vi "Save data.vi"(0 "Display State In":T2, 5 "Data":T1, 9 "Container State":T3, 11 "error in (no error)":errorcluster) -> (4 "Display State Out":T2, 15 "error out":errorcluster)   [LabVIEW 2014, in "Graph with cursors XControl.xctl"]
uses:
  Graph with cursors XControl.xctl
  <vilib>/_xctls/Container State.ctl
  Graph with cursors State.ctl
  Graph with cursors Data.ctl
  <vilib>/_xctls/XControlSupport.lvlib
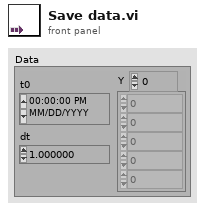
[diagram p1: front panel]
types:
  T1 = typedef "Graph with cursors XControl.xctl/Graph with cursors Data.ctl" = waveform(dbl)
  T2 = typedef "Graph with cursors XControl.xctl/Graph with cursors State.ctl" = cluster{"Cursor names":string[], "Cursor positions":dbl[], "Cursor pairs":i32, "Graph":refnum<vi>, "Prefix":string, "Base path":path}
  T3 = typedef "XControlSupport.lvlib/Container State.ctl" = cluster{"Indicator?":bool, "Run Mode?":bool, " Refnum":refnum<vi>}
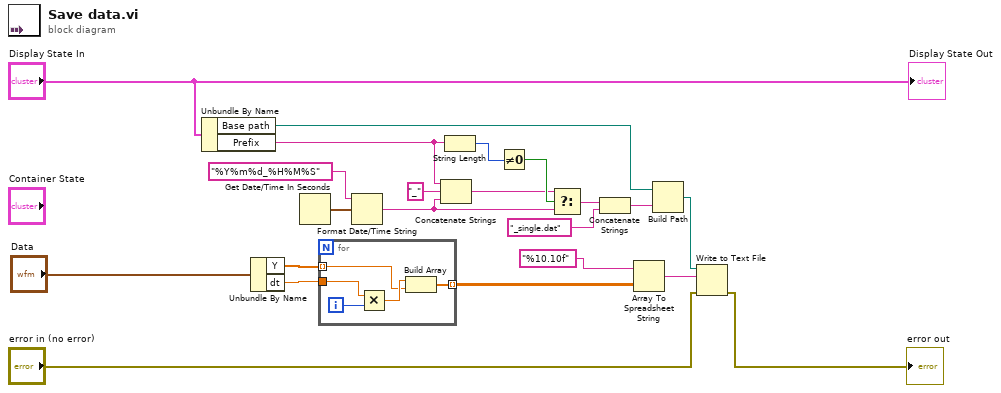
[diagram p0: block diagram]
diagram:
  n1 = Unbundle By Name("Display State In") -> ("Base path"=w11:path, "Prefix"=w10:string)
  n2 = Unbundle By Name("Data") -> ("Y"=w17:dbl[], "dt"=w16:dbl)
  n3 = Get Date/Time In Seconds() -> (seconds since 1Jan1904=w20:timestamp)
  n4 = for {
    tunnel: w17 -> [w24] mode=indexing
    tunnel: w16 -> [w26]
    tunnel: [w23] -> w1 mode=indexing
    i -> [w27]
    n5 = Multiply(x=w26, y=w27) -> (x*y=w25:dbl)
    n6 = Build Array(w25, w24) -> (w23:dbl[])
  }
  n7 = Format Date/Time String(time format string (%c)="%Y%m%d_%H%M%S", seconds (now)=w20) -> (date/time string=w7:string)  [unwired: 1 in]
  n8 = Concatenate Strings(w10, "_", w7) -> (w6:string)
  n9 = String Length(string=w10) -> (length=w9:i32)
  n10 = Not Equal To 0?(x=w9) -> (x != 0?=w8:bool)
  n11 = Select(t=w6, s=w8, f=w7) -> (s? t:f=w4:string)
  n12 = Concatenate Strings(w4, "_single.dat" ("string")) -> (w5:string)
  n13 = Array To Spreadsheet String(array=w1, 3:"%10.10f" ("format string")) -> (spreadsheet string=w15:string)  [unwired: 1 in]
  n14 = Build Path(base path=w11, name or relative path=w5) -> (appended path=w14:path)
  n15 = Write to Text File(file (use dialog)=w14, text=w15, error in="error in (no error)") -> (error out=→"error out":errorcluster)  [unwired: 1 in, 2 out]
  "Display State Out" <- "Display State In"
